vi "GUI_Bella_1BL.vi"() -> ()   [LabVIEW 2020]
uses:
  Shared/GUI_Template/GUI_master/tcp_new_data_event.ctl
  Shared/GUI_Template/GUI_master/tcp new data cluster.ctl
  <vilib>/vision/Image Controls.llb/IMAQ Image.ctl
  <vilib>/ErrorRing/Error Ring.xnode
panel:
  out "Display8":T1(plugin-control) caption="M1 Cam"
  in  "Target.X::8":dbl=0.001 caption="X" min=0.0 max=2000.0
  in  "Target.Y::8":dbl=0.001 caption="Y" min=0.0 max=2000.0
  in  "size8":dbl=20.0 caption="Size" min=0.0 max=0.0
  out "Display7":T1(plugin-control) caption="M1 Cam"
  in  "Target.X::7":dbl=0.001 caption="X" min=0.0 max=2000.0
  in  "Target.Y::7":dbl=0.001 caption="Y" min=0.0 max=2000.0
  in  "size7":dbl=20.0 caption="Size" min=0.0 max=0.0
  out "Display6":T1(plugin-control) caption="M1 Cam"
  in  "Target.X::6":dbl=0.001 caption="X" min=0.0 max=2000.0
  in  "Target.Y::6":dbl=0.001 caption="Y" min=0.0 max=2000.0
  in  "size6":dbl=20.0 caption="Size" min=0.0 max=0.0
  out "error out":errorcluster
  in  "GUIdevice 7":string="CAM-1BL-M5" caption="CAMERA 7"
  in  "GUIdevice 6":string="CAM-1BL-M2Near" caption="CAMERA 6"
  in  "GUIdevice 8":string="CAM-1BL-Ghost" caption="CAMERA 8"
  out "image::7":T1(plugin-control) caption="M1 Cam"
  out "image::8":T1(plugin-control) caption="M1 Cam"
  in  "centroidx::6":dbl=0.001 caption="X" min=0.0 max=0.0
  in  "centroidy::7":dbl=0.001 caption="Y" min=0.0 max=0.0
  in  "centroidx::7":dbl=0.001 caption="X" min=0.0 max=0.0
  in  "exposure::7":dbl=0.001 caption="Exposure" min=3.8e-05 max=1.0 format="%_4p"
  in  "trigger::7":bool caption="Blank Button"
  in  "centroidy::6":dbl=0.001 caption="Y" min=0.0 max=0.0
  in  "exposure::8":dbl=0.001 caption="Exposure" min=3.8e-05 max=1.0 format="%_4p"
  in  "trigger::8":bool caption="Blank Button"
  in  "centroidy::8":dbl=0.001 caption="Y" min=0.0 max=0.0
  in  "centroidx::8":dbl=0.001 caption="X" min=0.0 max=0.0
  in  "exposure::6":dbl=0.001 caption="Exposure" min=3.8e-05 max=1.0 format="%_4p"
  in  "trigger::6":bool caption="Blank Button"
  in  "image::6":T1(plugin-control) caption="M1 Cam"
  in  "roi::6":bool caption="Blank Button"
  in  "roi::7":bool caption="Blank Button"
  in  "roi::8":bool caption="Blank Button"
  out "Display5":T1(plugin-control) caption="M1 Cam"
  in  "Target.X::5":dbl=0.001 caption="X" min=0.0 max=2000.0
  in  "Target.Y::5":dbl=0.001 caption="Y" min=0.0 max=2000.0
  in  "size5":dbl=20.0 caption="Size" min=0.0 max=0.0
  out "Display4":T1(plugin-control) caption="M1 Cam"
  in  "Target.X::4":dbl=0.001 caption="X" min=0.0 max=2000.0
  in  "Target.Y::4":dbl=0.001 caption="Y" min=0.0 max=2000.0
  in  "size4":dbl=20.0 caption="Size" min=0.0 max=0.0
  out "Display3":T1(plugin-control) caption="M1 Cam"
  in  "Target.X::3":dbl=0.001 caption="X" min=0.0 max=2000.0
  in  "Target.Y::3":dbl=0.001 caption="Y" min=0.0 max=2000.0
  in  "size3":dbl=20.0 caption="Size" min=0.0 max=0.0
  in  "Target.X::2":dbl=0.001 caption="X" min=0.0 max=2000.0
  in  "Target.Y::2":dbl=0.001 caption="Y" min=0.0 max=2000.0
  in  "size2":dbl=20.0 caption="Size" min=0.0 max=0.0
  out "Display2":T1(plugin-control) caption="M1 Cam"
  in  "roi::5":bool caption="Blank Button"
  in  "centroidx::5":dbl=0.001 caption="X" min=0.0 max=0.0
  in  "centroidy::5":dbl=0.001 caption="Y" min=0.0 max=0.0
  in  "trigger::5":bool caption="Blank Button"
  in  "exposure::5":dbl=0.001 caption="Exposure" min=3.8e-05 max=1.0 format="%_4p"
  in  "GUIdevice 5":string="CAM-1BL-M1" caption="CAMERA 5"
  in  "roi::4":bool caption="Blank Button"
  in  "centroidx::4":dbl=0.001 caption="X" min=0.0 max=0.0
  in  "centroidy::4":dbl=0.001 caption="Y" min=0.0 max=0.0
  in  "trigger::4":bool caption="Blank Button"
  in  "exposure::4":dbl=0.001 caption="Exposure" min=3.8e-05 max=1.0 format="%_4p"
  in  "GUIdevice 4":string="CAM-LT-Comp-IN" caption="CAMERA 4"
  in  "roi::3":bool caption="Blank Button"
  in  "centroidx::3":dbl=0.001 caption="X" min=0.0 max=0.0
  in  "centroidy::3":dbl=0.001 caption="Y" min=0.0 max=0.0
  in  "trigger::3":bool caption="Blank Button"
  in  "exposure::3":dbl=0.001 caption="Exposure" min=3.8e-05 max=1.0 format="%_4p"
  in  "GUIdevice 3":string="CAM-1BL-ShotControl" caption="CAMERA 3"
  in  "roi::1":bool caption="Blank Button"
  in  "size1":dbl=20.0 caption="Size" min=0.0 max=0.0
  in  "Target.X::1":dbl=0.001 caption="X" min=0.0 max=2000.0
  in  "Target.Y::1":dbl=0.001 caption="Y" min=0.0 max=2000.0
  in  "centroidx::1":dbl=0.001 caption="X" min=0.0 max=0.0
  in  "centroidy::1":dbl=0.001 caption="Y" min=0.0 max=0.0
  in  "trigger::1":bool caption="Blank Button"
  in  "exposure::1":dbl=0.001 caption="Exposure" min=3.8e-05 max=1.0 format="%_4p"
  in  "GUIdevice 1":string="CAM-LT-Amp3Leak" caption="CAMERA 1"
  out "Display1":T1(plugin-control) caption="M1 Cam"
  in  "roi::2":bool caption="Blank Button"
  in  "centroidx::2":dbl=0.001 caption="X" min=0.0 max=0.0
  in  "centroidy::2":dbl=0.001 caption="Y" min=0.0 max=0.0
  in  "trigger::2":bool caption="Blank Button"
  in  "exposure::2":dbl=0.001 caption="Exposure" min=3.8e-05 max=1.0 format="%_4p"
  in  "GUIdevice 2":string="CAM-1BL-DM" caption="CAMERA 2"
  out "image::5":T1(plugin-control) caption="M1 Cam"
  out "image::4":T1(plugin-control) caption="M1 Cam"
  in  "image::3":T1(plugin-control) caption="M1 Cam"
  out "image::2":T1(plugin-control) caption="M1 Cam"
  out "image::1":T1(plugin-control) caption="M1 Cam"
  out "tcp data event":T2
  in  "stop":bool
  out "error IO 2":errorcluster
  # "1BL GUI - 1"
  # "Target"
  # "Centroid"
  # "Target"
  # "Centroid"
  # "Target"
  # "Target"
  # "Centroid"
  # "Centroid"
  # "Target"
  # "Target"
  # "Target"
  # "Centroid"
  # "Centroid"
  # "Centroid"
  # "Target"
  # "Centroid"
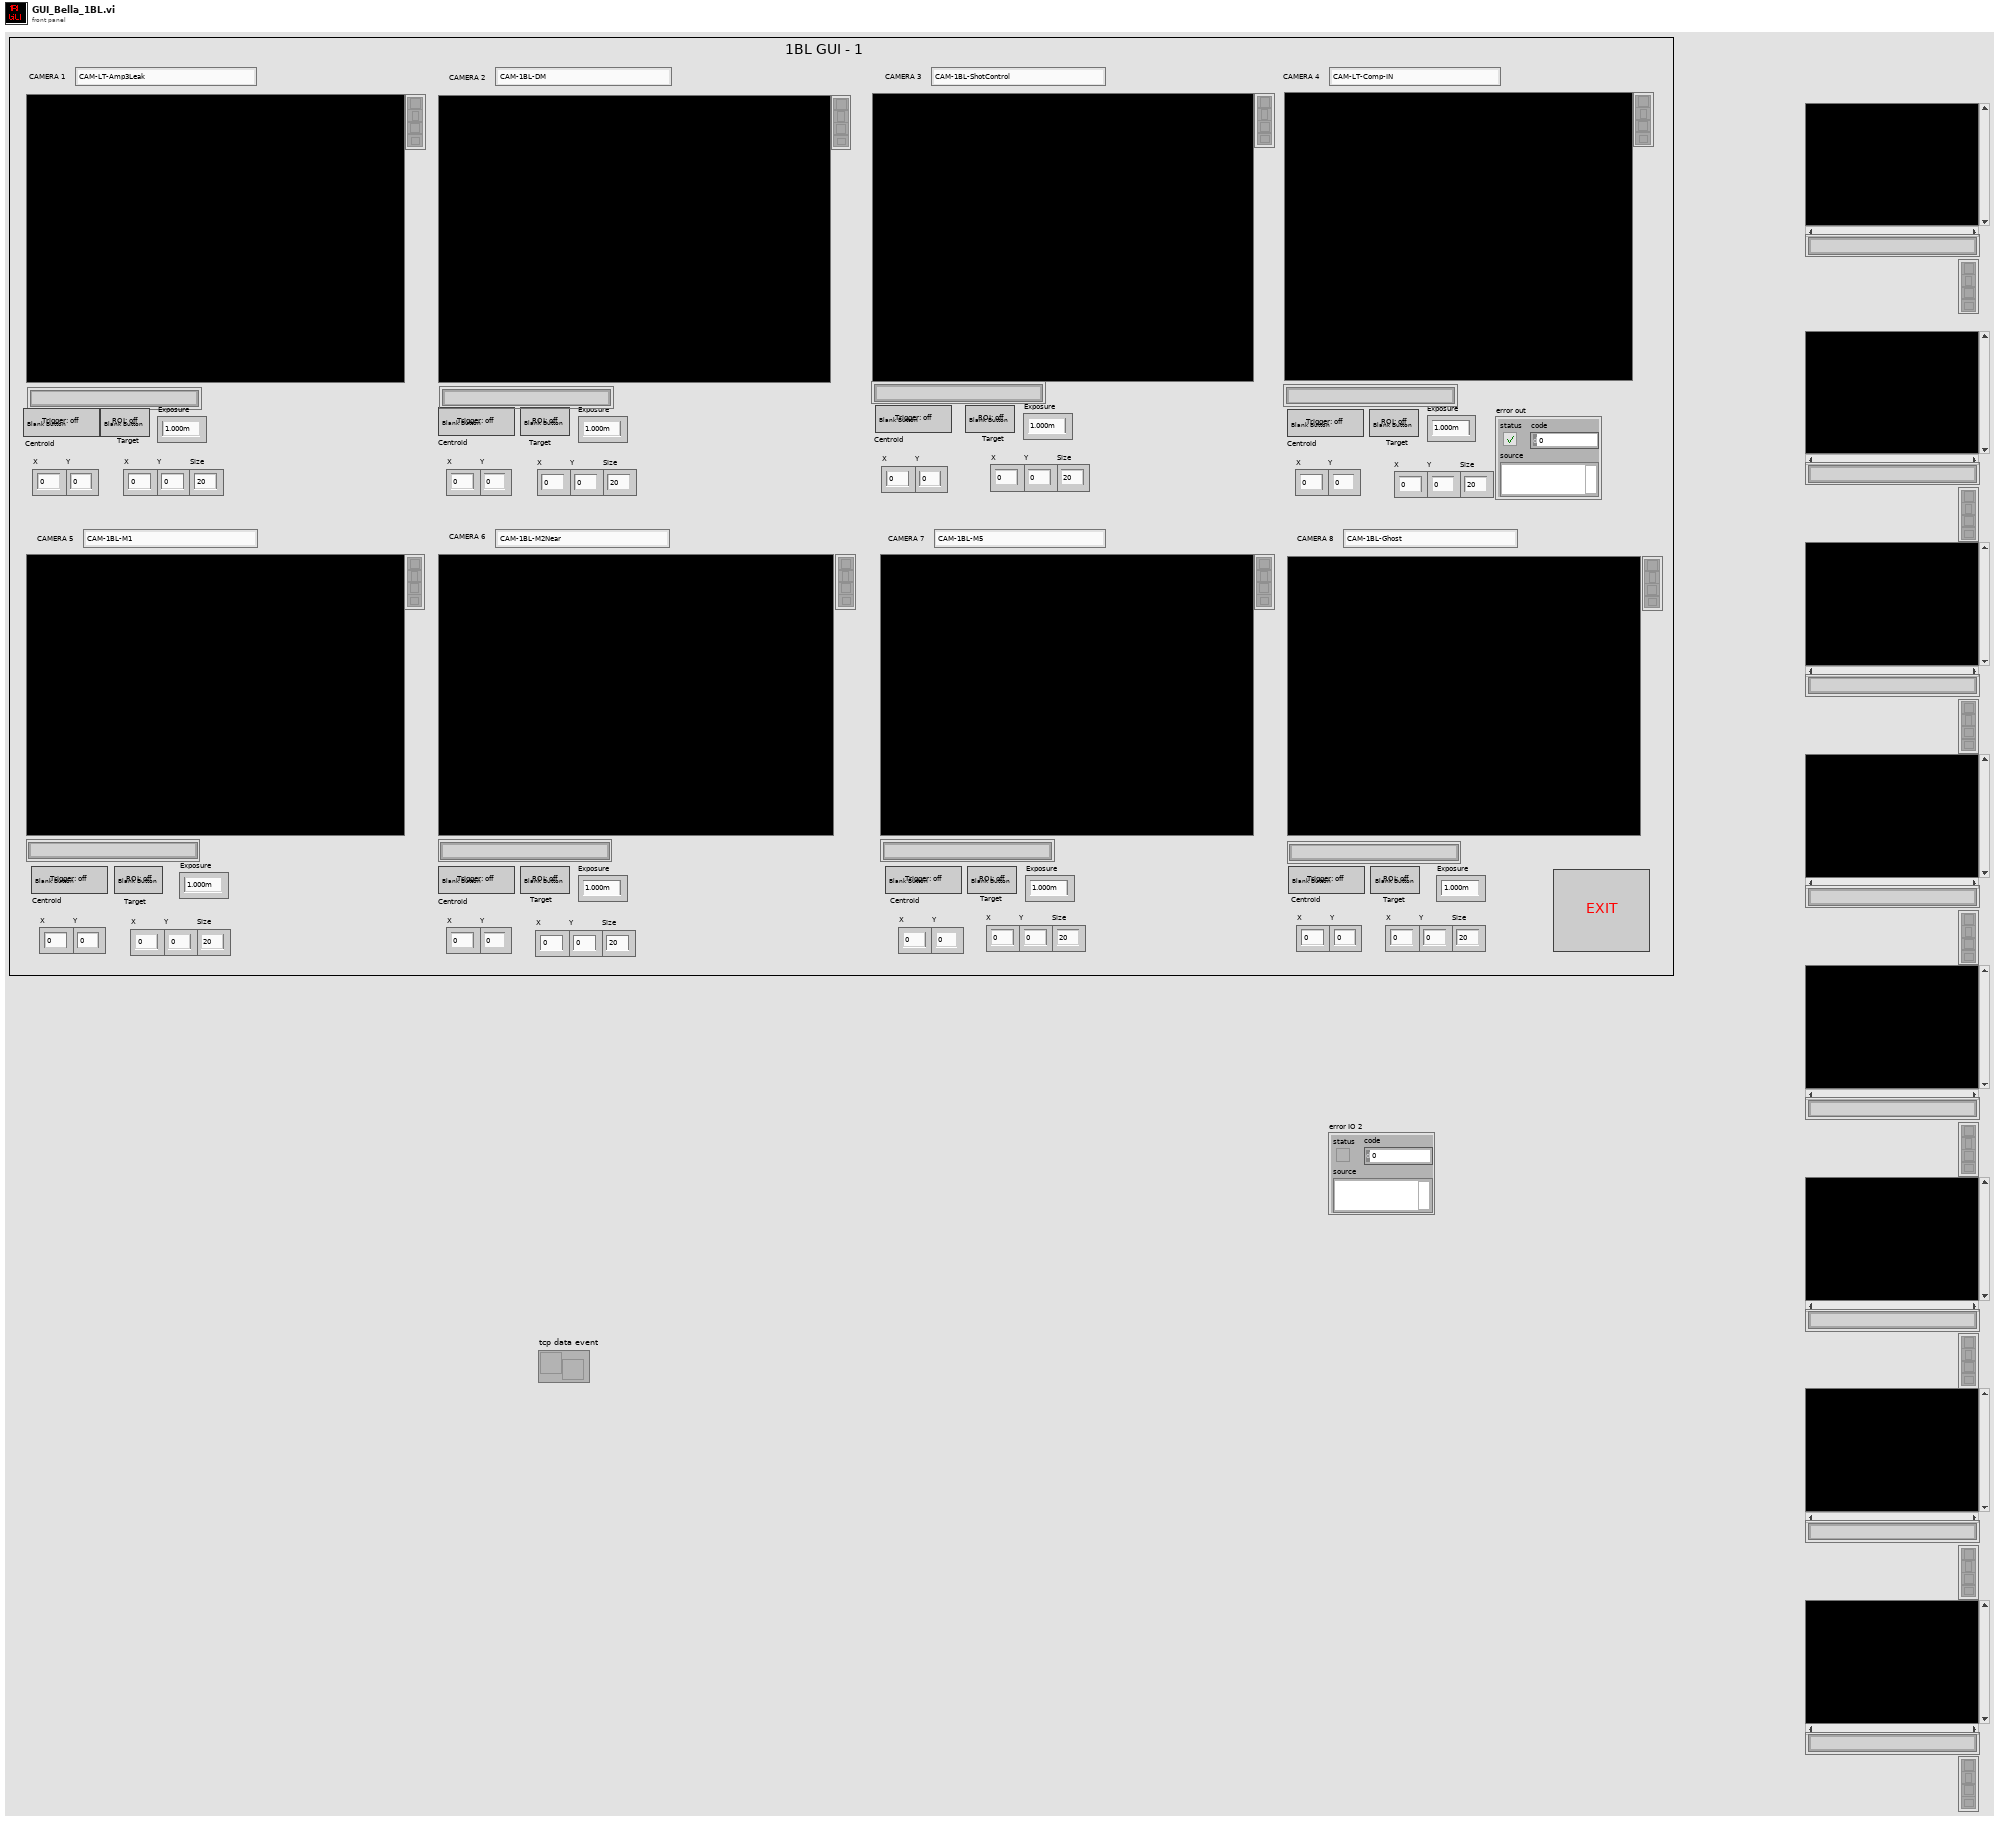
[diagram p1: front panel]
types:
  T1 = typedef "IMAQ Image.ctl" = refnum<image>
  T2 = typedef "tcp_new_data_event.ctl" = refnum<user-event>
  T3 = cluster{"Image1":T1, "Image2":T1, "Image3":T1, "Image4":T1, "Image5":T1, "Image6":T1, "Image7":T1, "Image8":T1}
  T4 = cluster{"Last update Cam1":u32, "Last update Cam2":u32, "Last update Cam3":u32, "Last update Cam4":u32, "Last update Cam5":u32, "Last update Cam6":u32, "Last update Cam7":u32, "Last update Cam8":u32}
  T5 = typedef "Image Type" = u32
  T6 = typedef "tcp new data cluster.ctl" = cluster{"EventEnum":enum16{"new data", "connection status update"}, "Device name":string}
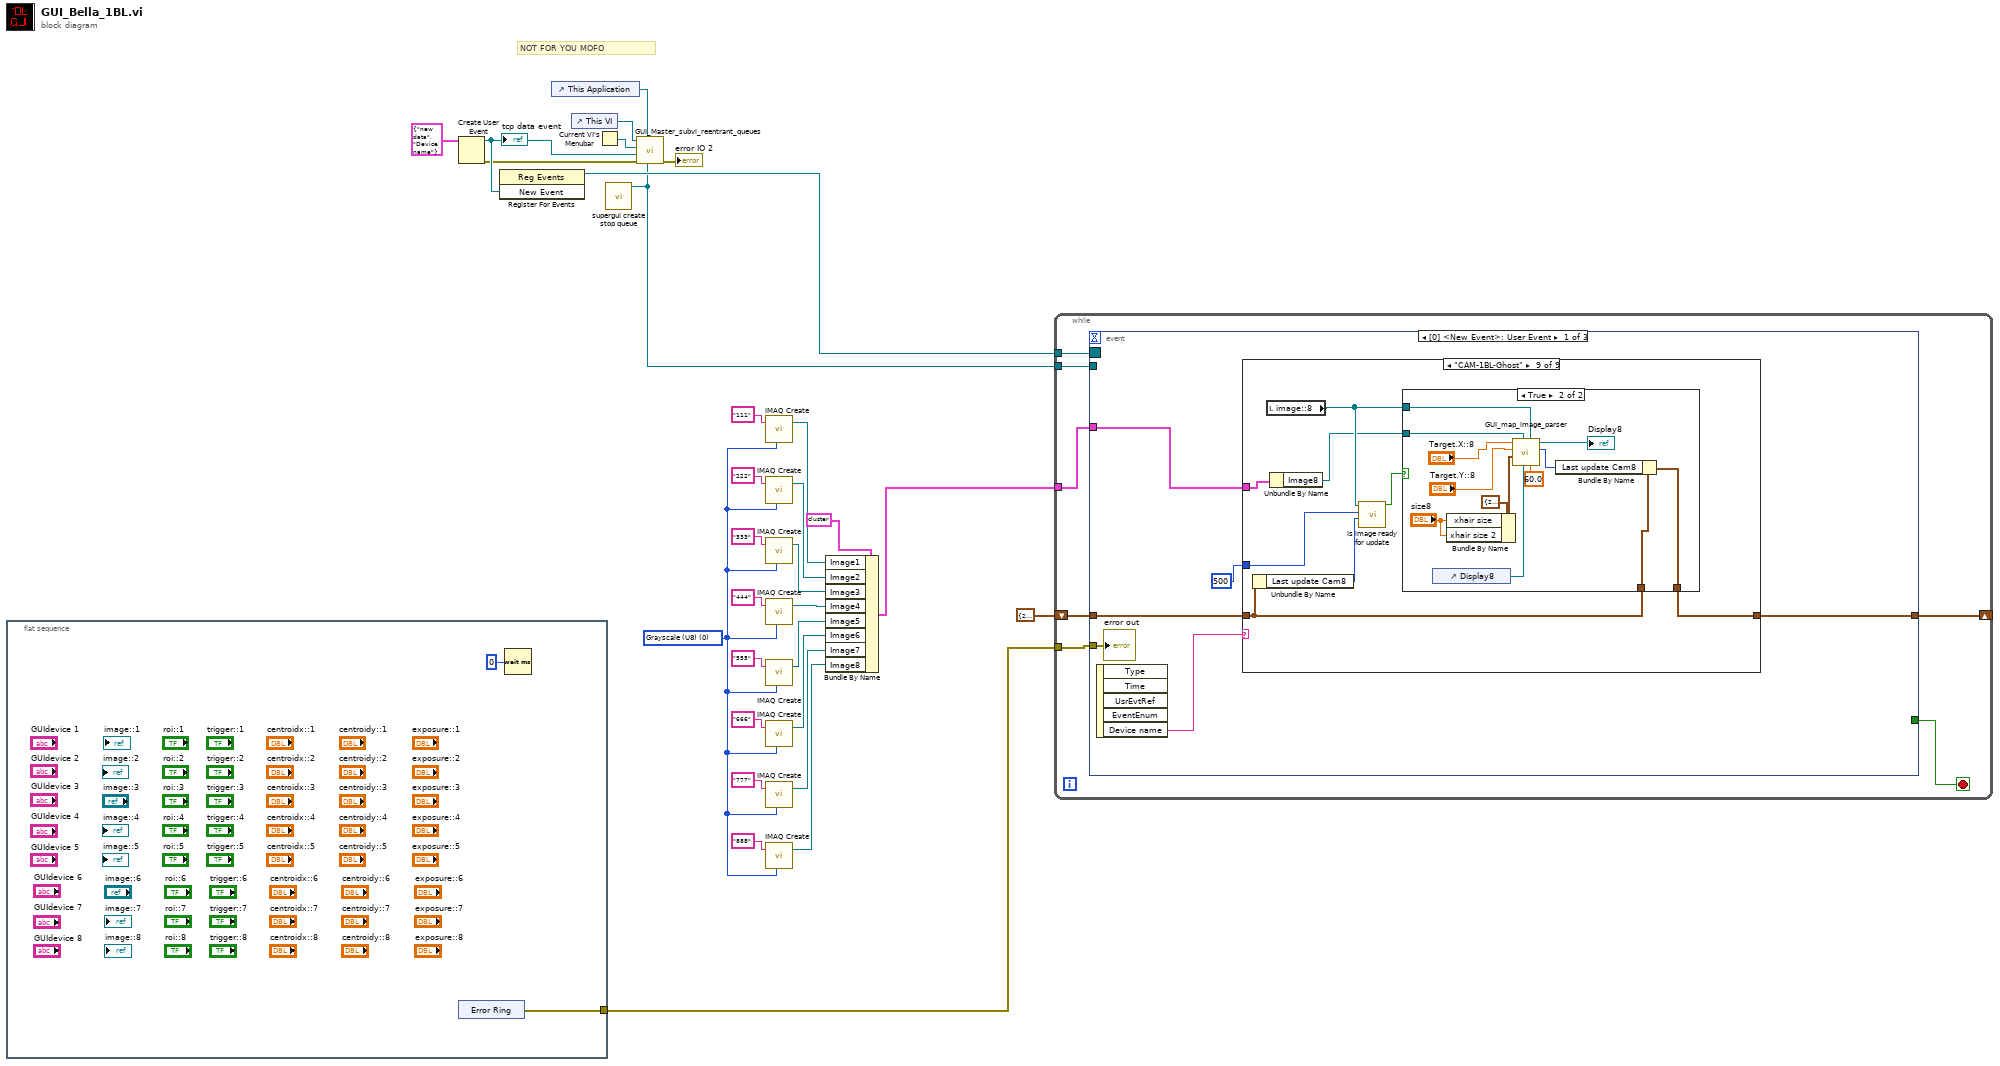
[diagram p0: block diagram]
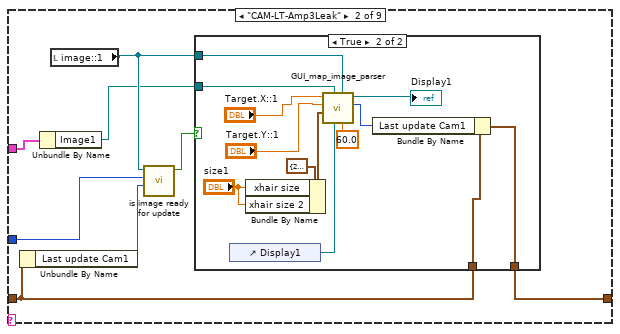
[diagram p3: hidden frame]
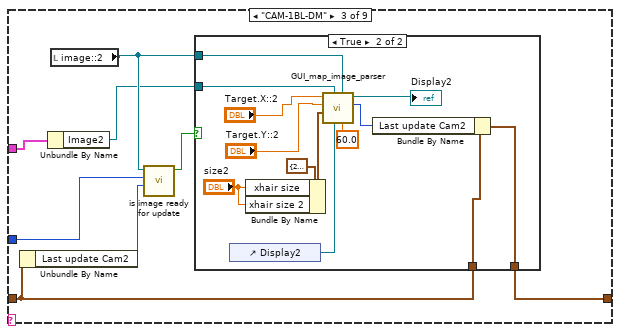
[diagram p5: hidden frame]
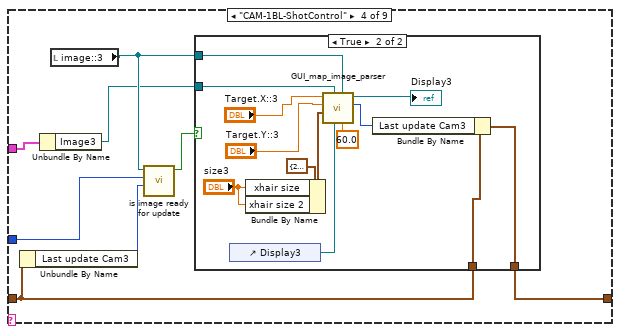
[diagram p7: hidden frame]
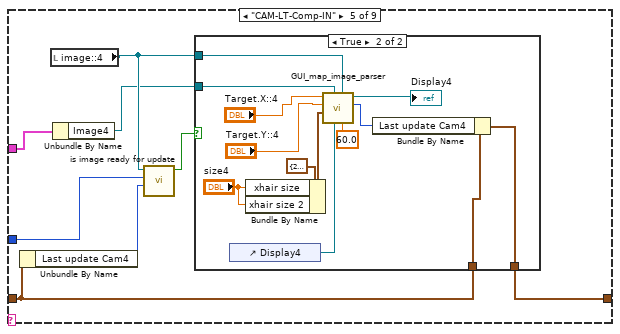
[diagram p9: hidden frame]
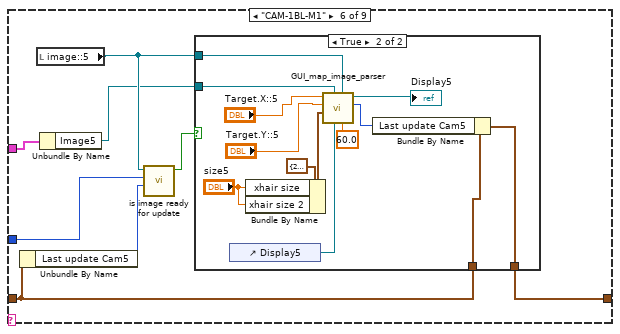
[diagram p11: hidden frame]
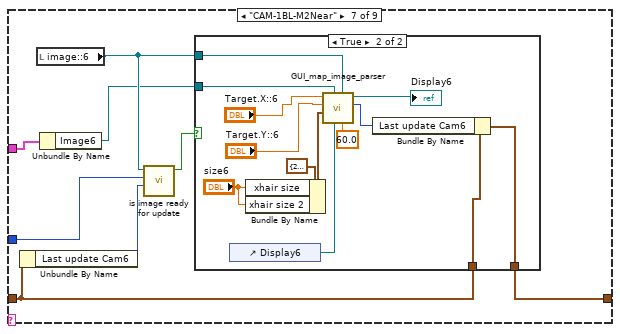
[diagram p13: hidden frame]
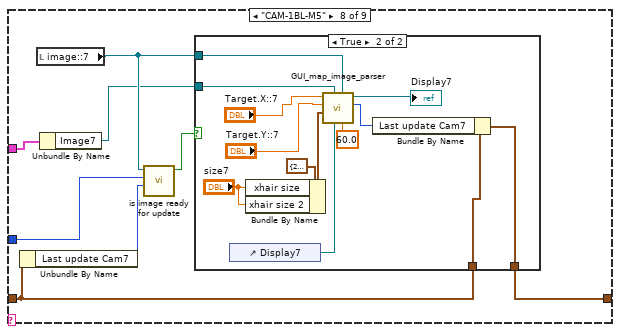
[diagram p15: hidden frame]
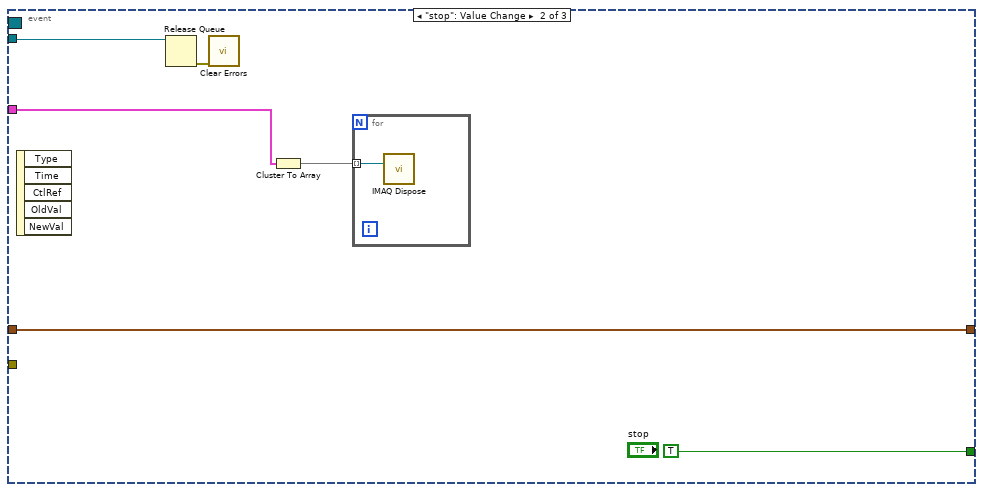
[diagram p18: hidden frame]
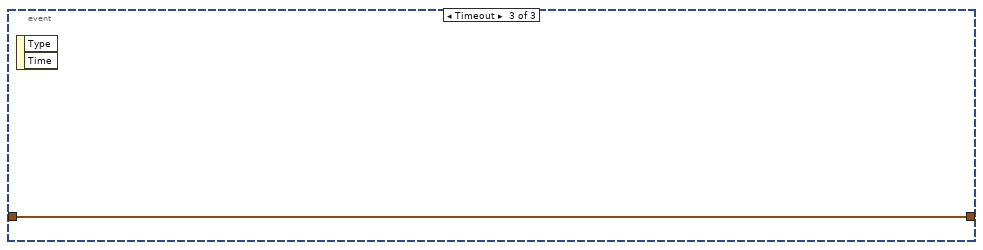
[diagram p19: hidden frame]
diagram:
  w12 = T5 0 items=["Grayscale (U8)", "Grayscale (I16)", "Grayscale (SGL)", "Complex (CSG)", "RGB (U32)", "HSL (U32)", "RGB (U64)", "Grayscale (U16)"] ("Image Type")
  # "NOT FOR YOU MOFO"
  n1 = flat-sequence {
    tunnel: [w32] -> w1
    frame #0 {
      n2 = xnode "Error Ring"() -> ("error out"=w32:errorcluster)
      n3 = Wait (ms)(milliseconds to wait=u32 0) -> ()  [unwired: 1 out]
    }
  }
  n4 = Create User Event(user event datatype=T6 {"EventEnum"=enum."new data", "Device name"="Device name"} ("New Event")) -> (user event=w29:refnum<user-event>, error out=w28:errorcluster)  [unwired: 1 in]
  "tcp data event" <- w29
  n5 = register-events(w29) -> (reference out=w24:refnum<event-registration>)  [unwired: 2 in, 1 out]
  n6 = control-ref of="This Application"() -> (w30:refnum<vi>)
  n7 = control-ref of="This VI"() -> (w25:refnum<vi>)
  n8 = Current VI's Menubar() -> (w26:refnum<k9>)
  n9 = call "supergui create stop queue.vi"() -> ("STOP Queue out"=w16:refnum<queue>)  [unwired: 11 in]
  n10 = call "GUI_Master_subvi_reentrant_queues.vi"("STOP Queue in"=w16, "This Application"=w30, "error in (no error)"=w28, "tcp data event"=w29, "Caller menu reference"=w26, "Caller VI ref"=w25) -> ("error out"=→"error IO 2":errorcluster)  [unwired: 5 in]
  n11 = call "IMAQ Create"("Image Name"="111", "Image Type"=w12) -> ("New Image"=w11:T1)  [unwired: 3 in, 1 out]
  n12 = call "IMAQ Create"("Image Name"="222", "Image Type"=w12) -> ("New Image"=w10:T1)  [unwired: 3 in, 1 out]
  n13 = call "IMAQ Create"("Image Name"="333", "Image Type"=w12) -> ("New Image"=w9:T1)  [unwired: 3 in, 1 out]
  n14 = call "IMAQ Create"("Image Name"="444", "Image Type"=w12) -> ("New Image"=w8:T1)  [unwired: 3 in, 1 out]
  n15 = call "IMAQ Create"("Image Name"="555", "Image Type"=w12) -> ("New Image"=w7:T1)  [unwired: 3 in, 1 out]
  n16 = call "IMAQ Create"("Image Name"="666", "Image Type"=w12) -> ("New Image"=w6:T1)  [unwired: 3 in, 1 out]
  n17 = call "IMAQ Create"("Image Name"="777", "Image Type"=w12) -> ("New Image"=w5:T1)  [unwired: 3 in, 1 out]
  n18 = call "IMAQ Create"("Image Name"="888", "Image Type"=w12) -> ("New Image"=w4:T1)  [unwired: 3 in, 1 out]
  n19 = Bundle By Name(cluster=T3 {"Image1"=refnum, "Image2"=refnum, "Image3"=refnum, "Image4"=refnum, "Image5"=refnum, "Image6"=refnum, "Image7"=refnum, "Image8"=refnum}, "Image1"=w11, "Image2"=w10, "Image3"=w9, "Image4"=w8, "Image5"=w7, "Image6"=w6, "Image7"=w5, "Image8"=w4) -> (w2:T3)
  n20 = while {
    tunnel: w24 -> [w39]
    shift-right: [w37] -> _
    shift-left: T4 {"Last update Cam1"=200, "Last update Cam2"=200, "Last update Cam3"=200, "Last update Cam4"=200, "Last update Cam5"=200, "Last update Cam6"=200, "Last update Cam7"=200, "Last update Cam8"=200} -> [w38]
    tunnel: w16 -> [w36]
    tunnel: w2 -> [w35]
    tunnel: w1 -> [w34]
    stop <- w40 stop-if-true
    n21 = event shown="[0] <New Event>: User Event" {
      selector: w39 -> [_ _ _]
      dyn-events: _ -> [_ _ _]
      timeout: _ -> [_ _ _]
      tunnel: [_ TRUE ("stop") _] -> w40
      tunnel: w38 -> [w45 w228 w231]
      tunnel: [w43 w228 w231] -> w37
      tunnel: w36 -> [_ w227 _]
      tunnel: w35 -> [w42 w225 _]
      tunnel: w34 -> [w41 _ _]
      event User Event {
        n22 = event-data() -> ("Device name"=w46:string)  [unwired: 1 in, 4 out]
        n23 = case shown="\"CAM-1BL-Ghost\"" w46 {
          tunnel: w45 -> [w47 w55 w77 w99 w121 w143 w165 w187 w209]
          tunnel: u32 500 ("x-y") -> [_ w53 w75 w97 w119 w141 w163 w185 w207]
          tunnel: [w47 w54 w76 w98 w120 w142 w164 w186 w208] -> w43
          tunnel: w42 -> [_ w49 w71 w93 w115 w137 w159 w181 w203]
          frame Default {
          }
          frame "CAM-LT-Amp3Leak" {
            n24 = Unbundle By Name(w55) -> ("Last update Cam1"=w52:u32)
            n25 = Unbundle By Name(w49) -> ("Image1"=w48:T1)
            n26 = local read "image::1"() -> (w50:T1)
            n27 = call "is image ready for update.vi"("Last update"=w52, "min time between updates"=w53, "image ref in"=w50) -> ("update image"=w51:bool)  [unwired: 8 in]
            n28 = case shown="True" w51 {
              tunnel: w55 -> [w56 w69]
              tunnel: [w56 w68] -> w54
              tunnel: w50 -> [_ w67]
              tunnel: w48 -> [_ w57]
              frame False {
              }
              frame True {
                n29 = control-ref of="Display1"() -> (w63:refnum<vi>)
                n30 = Bundle By Name(cluster=cluster{"xhair size":dbl, "xhair size 2":dbl} {"xhair size"=20.0, "xhair size 2"=20.0} ("size"), "xhair size"="size1", "xhair size 2"="size1") -> (w58:cluster{"xhair size":dbl, "xhair size 2":dbl})
                n31 = call "GUI_map_image_parser.vi"("zoom#"=60.0, "Image Src"=w67, "Ctl Refnum"=w63, "Image Dst"=w57, "size"=w58, "target y"="Target.Y::1", "target x"="Target.X::1") -> ("ms timer out"=w62:u32, "Img out"=→"Display1":T1)  [unwired: 3 in]
                n32 = Bundle By Name(cluster=w69, "Last update Cam1"=w62) -> (w68:T4)
              }
            }
          }
          frame "CAM-1BL-DM" {
            n33 = Unbundle By Name(w77) -> ("Last update Cam2"=w74:u32)
            n34 = Unbundle By Name(w71) -> ("Image2"=w70:T1)
            n35 = local read "image::2"() -> (w72:T1)
            n36 = call "is image ready for update.vi"("Last update"=w74, "min time between updates"=w75, "image ref in"=w72) -> ("update image"=w73:bool)  [unwired: 8 in]
            n37 = case shown="True" w73 {
              tunnel: w77 -> [w78 w91]
              tunnel: [w78 w90] -> w76
              tunnel: w72 -> [_ w89]
              tunnel: w70 -> [_ w79]
              frame False {
              }
              frame True {
                n38 = control-ref of="Display2"() -> (w85:refnum<vi>)
                n39 = Bundle By Name(cluster=cluster{"xhair size":dbl, "xhair size 2":dbl} {"xhair size"=20.0, "xhair size 2"=20.0} ("size"), "xhair size"="size2", "xhair size 2"="size2") -> (w80:cluster{"xhair size":dbl, "xhair size 2":dbl})
                n40 = call "GUI_map_image_parser.vi"("zoom#"=60.0, "Image Src"=w89, "Ctl Refnum"=w85, "Image Dst"=w79, "size"=w80, "target y"="Target.Y::2", "target x"="Target.X::2") -> ("ms timer out"=w84:u32, "Img out"=→"Display2":T1)  [unwired: 3 in]
                n41 = Bundle By Name(cluster=w91, "Last update Cam2"=w84) -> (w90:T4)
              }
            }
          }
          frame "CAM-1BL-ShotControl" {
            n42 = Unbundle By Name(w99) -> ("Last update Cam3"=w96:u32)
            n43 = Unbundle By Name(w93) -> ("Image3"=w92:T1)
            n44 = local read "image::3"() -> (w94:T1)
            n45 = call "is image ready for update.vi"("Last update"=w96, "min time between updates"=w97, "image ref in"=w94) -> ("update image"=w95:bool)  [unwired: 8 in]
            n46 = case shown="True" w95 {
              tunnel: w99 -> [w100 w113]
              tunnel: [w100 w112] -> w98
              tunnel: w94 -> [_ w111]
              tunnel: w92 -> [_ w101]
              frame False {
              }
              frame True {
                n47 = control-ref of="Display3"() -> (w107:refnum<vi>)
                n48 = Bundle By Name(cluster=cluster{"xhair size":dbl, "xhair size 2":dbl} {"xhair size"=20.0, "xhair size 2"=20.0} ("size"), "xhair size"="size3", "xhair size 2"="size3") -> (w102:cluster{"xhair size":dbl, "xhair size 2":dbl})
                n49 = call "GUI_map_image_parser.vi"("zoom#"=60.0, "Image Src"=w111, "Ctl Refnum"=w107, "Image Dst"=w101, "size"=w102, "target y"="Target.Y::3", "target x"="Target.X::3") -> ("ms timer out"=w106:u32, "Img out"=→"Display3":T1)  [unwired: 3 in]
                n50 = Bundle By Name(cluster=w113, "Last update Cam3"=w106) -> (w112:T4)
              }
            }
          }
          frame "CAM-LT-Comp-IN" {
            n51 = Unbundle By Name(w121) -> ("Last update Cam4"=w118:u32)
            n52 = local read "image::4"() -> (w116:T1)
            n53 = Unbundle By Name(w115) -> ("Image4"=w114:T1)
            n54 = call "is image ready for update.vi"("Last update"=w118, "min time between updates"=w119, "image ref in"=w116) -> ("update image"=w117:bool)  [unwired: 8 in]
            n55 = case shown="True" w117 {
              tunnel: w121 -> [w122 w135]
              tunnel: [w122 w134] -> w120
              tunnel: w116 -> [_ w133]
              tunnel: w114 -> [_ w123]
              frame False {
              }
              frame True {
                n56 = control-ref of="Display4"() -> (w129:refnum<vi>)
                n57 = Bundle By Name(cluster=cluster{"xhair size":dbl, "xhair size 2":dbl} {"xhair size"=20.0, "xhair size 2"=20.0} ("size"), "xhair size"="size4", "xhair size 2"="size4") -> (w124:cluster{"xhair size":dbl, "xhair size 2":dbl})
                n58 = call "GUI_map_image_parser.vi"("zoom#"=60.0, "Image Src"=w133, "Ctl Refnum"=w129, "Image Dst"=w123, "size"=w124, "target y"="Target.Y::4", "target x"="Target.X::4") -> ("ms timer out"=w128:u32, "Img out"=→"Display4":T1)  [unwired: 3 in]
                n59 = Bundle By Name(cluster=w135, "Last update Cam4"=w128) -> (w134:T4)
              }
            }
          }
          frame "CAM-1BL-M1" {
            n60 = Unbundle By Name(w143) -> ("Last update Cam5"=w140:u32)
            n61 = local read "image::5"() -> (w138:T1)
            n62 = Unbundle By Name(w137) -> ("Image5"=w136:T1)
            n63 = call "is image ready for update.vi"("Last update"=w140, "min time between updates"=w141, "image ref in"=w138) -> ("update image"=w139:bool)  [unwired: 8 in]
            n64 = case shown="True" w139 {
              tunnel: w143 -> [w144 w157]
              tunnel: [w144 w156] -> w142
              tunnel: w138 -> [_ w155]
              tunnel: w136 -> [_ w145]
              frame False {
              }
              frame True {
                n65 = control-ref of="Display5"() -> (w151:refnum<vi>)
                n66 = Bundle By Name(cluster=cluster{"xhair size":dbl, "xhair size 2":dbl} {"xhair size"=20.0, "xhair size 2"=20.0} ("size"), "xhair size"="size5", "xhair size 2"="size5") -> (w146:cluster{"xhair size":dbl, "xhair size 2":dbl})
                n67 = call "GUI_map_image_parser.vi"("zoom#"=60.0, "Image Src"=w155, "Ctl Refnum"=w151, "Image Dst"=w145, "size"=w146, "target y"="Target.Y::5", "target x"="Target.X::5") -> ("ms timer out"=w150:u32, "Img out"=→"Display5":T1)  [unwired: 3 in]
                n68 = Bundle By Name(cluster=w157, "Last update Cam5"=w150) -> (w156:T4)
              }
            }
          }
          frame "CAM-1BL-M2Near" {
            n69 = Unbundle By Name(w165) -> ("Last update Cam6"=w162:u32)
            n70 = local read "image::6"() -> (w160:T1)
            n71 = Unbundle By Name(w159) -> ("Image6"=w158:T1)
            n72 = call "is image ready for update.vi"("Last update"=w162, "min time between updates"=w163, "image ref in"=w160) -> ("update image"=w161:bool)  [unwired: 8 in]
            n73 = case shown="True" w161 {
              tunnel: w165 -> [w166 w179]
              tunnel: [w166 w178] -> w164
              tunnel: w160 -> [_ w177]
              tunnel: w158 -> [_ w167]
              frame False {
              }
              frame True {
                n74 = control-ref of="Display6"() -> (w173:refnum<vi>)
                n75 = Bundle By Name(cluster=cluster{"xhair size":dbl, "xhair size 2":dbl} {"xhair size"=20.0, "xhair size 2"=20.0} ("size"), "xhair size"="size6", "xhair size 2"="size6") -> (w168:cluster{"xhair size":dbl, "xhair size 2":dbl})
                n76 = call "GUI_map_image_parser.vi"("zoom#"=60.0, "Image Src"=w177, "Ctl Refnum"=w173, "Image Dst"=w167, "size"=w168, "target y"="Target.Y::6", "target x"="Target.X::6") -> ("ms timer out"=w172:u32, "Img out"=→"Display6":T1)  [unwired: 3 in]
                n77 = Bundle By Name(cluster=w179, "Last update Cam6"=w172) -> (w178:T4)
              }
            }
          }
          frame "CAM-1BL-M5" {
            n78 = Unbundle By Name(w187) -> ("Last update Cam7"=w184:u32)
            n79 = local read "image::7"() -> (w182:T1)
            n80 = Unbundle By Name(w181) -> ("Image7"=w180:T1)
            n81 = call "is image ready for update.vi"("Last update"=w184, "min time between updates"=w185, "image ref in"=w182) -> ("update image"=w183:bool)  [unwired: 8 in]
            n82 = case shown="True" w183 {
              tunnel: w187 -> [w188 w201]
              tunnel: [w188 w200] -> w186
              tunnel: w182 -> [_ w199]
              tunnel: w180 -> [_ w189]
              frame False {
              }
              frame True {
                n83 = control-ref of="Display7"() -> (w195:refnum<vi>)
                n84 = Bundle By Name(cluster=cluster{"xhair size":dbl, "xhair size 2":dbl} {"xhair size"=20.0, "xhair size 2"=20.0} ("size"), "xhair size"="size7", "xhair size 2"="size7") -> (w190:cluster{"xhair size":dbl, "xhair size 2":dbl})
                n85 = call "GUI_map_image_parser.vi"("zoom#"=60.0, "Image Src"=w199, "Ctl Refnum"=w195, "Image Dst"=w189, "size"=w190, "target y"="Target.Y::7", "target x"="Target.X::7") -> ("ms timer out"=w194:u32, "Img out"=→"Display7":T1)  [unwired: 3 in]
                n86 = Bundle By Name(cluster=w201, "Last update Cam7"=w194) -> (w200:T4)
              }
            }
          }
          frame "CAM-1BL-Ghost" {
            n87 = Unbundle By Name(w209) -> ("Last update Cam8"=w206:u32)
            n88 = local read "image::8"() -> (w204:T1)
            n89 = Unbundle By Name(w203) -> ("Image8"=w202:T1)
            n90 = call "is image ready for update.vi"("Last update"=w206, "min time between updates"=w207, "image ref in"=w204) -> ("update image"=w205:bool)  [unwired: 8 in]
            n91 = case shown="True" w205 {
              tunnel: w209 -> [w210 w223]
              tunnel: [w210 w222] -> w208
              tunnel: w204 -> [_ w221]
              tunnel: w202 -> [_ w211]
              frame False {
              }
              frame True {
                n92 = control-ref of="Display8"() -> (w217:refnum<vi>)
                n93 = Bundle By Name(cluster=cluster{"xhair size":dbl, "xhair size 2":dbl} {"xhair size"=20.0, "xhair size 2"=20.0} ("size"), "xhair size"="size8", "xhair size 2"="size8") -> (w212:cluster{"xhair size":dbl, "xhair size 2":dbl})
                n94 = call "GUI_map_image_parser.vi"("zoom#"=60.0, "Image Src"=w221, "Ctl Refnum"=w217, "Image Dst"=w211, "size"=w212, "target y"="Target.Y::8", "target x"="Target.X::8") -> ("ms timer out"=w216:u32, "Img out"=→"Display8":T1)  [unwired: 3 in]
                n95 = Bundle By Name(cluster=w223, "Last update Cam8"=w216) -> (w222:T4)
              }
            }
          }
        }
        "error out" <- w41
      }
      event "stop": Value Change {
        n96 = event-data() -> ()  [unwired: 1 in, 5 out]
        n97 = Release Queue(queue=w227) -> (error out=w226:errorcluster)  [unwired: 2 in, 2 out]
        n98 = call <vilib>:"Clear Errors.vi"("error in (no error)"=w226) -> ()  [unwired: 5 in, 2 out]
        n99 = Cluster To Array(cluster=w225) -> (array=w224:T1[])
        n100 = for {
          tunnel: w224 -> [w230] mode=indexing
          n101 = call "IMAQ Dispose"("Image"=w230) -> ()  [unwired: 5 in, 1 out]
        }
      }
      event Timeout {
        n102 = event-data() -> ()  [unwired: 1 in, 2 out]
      }
    }
  }
